vi "Transform Points using Homography Matrix.vi"(10 "Homography Matrix":dbl[][](array[numeric]), 11 "Points":cluster{"X":dbl, "Y":dbl}[](array[cluster])) -> (3 "Transformed Points":cluster{"X":dbl, "Y":dbl}[](array[cluster]))   [LabVIEW 2016]
doc: "The VI transforms the given array of points using the homography matrix.\n[x'] = [H] * [x]"
uses:
  <vilib>/Analysis/baseanly.llb/A x Vector.vi
  <vilib>/Analysis/NI_AALBase.lvlib
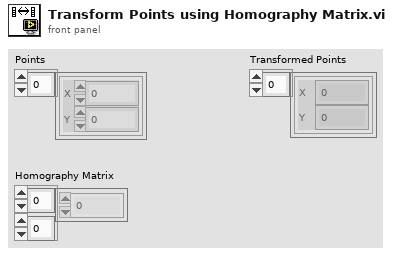
[diagram p1: front panel]
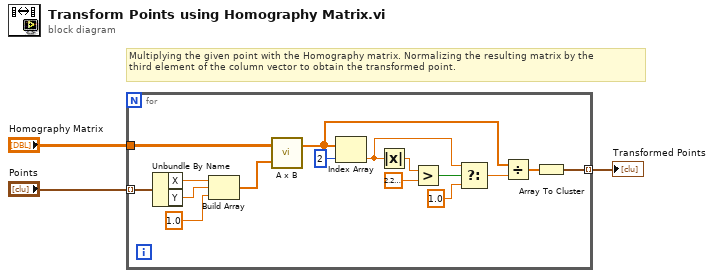
[diagram p0: block diagram]
diagram:
  # "Multiplying the given point with the Homography matrix. Normalizing the resulting matrix by the \nthird element of the column vector to obtain the transformed point."
  n1 = for {
    tunnel: "Homography Matrix" -> [w19]
    tunnel: "Points" -> [w12] mode=indexing
    tunnel: [w4] -> w2 mode=indexing
    n2 = Unbundle By Name(w12) -> ("X"=w11:dbl, "Y"=w10:dbl)
    n3 = Build Array(w11, w10, 1.0) -> (w13:dbl[])
    n4 = call-poly <vilib>:"A x B.vi"("Vector"=w13, "A"=w19) -> ("A x Vector"=w16:dbl[])  [unwired: 1 out]
    n5 = Index Array(array=w16, index=2) -> (element=w8:dbl)
    n6 = Absolute Value(x=w8) -> (abs(x)=w17:dbl)
    n7 = Greater?(x=w17, y=2.220446049250313e-16) -> (0:w9:bool)
    n8 = Select(t=w8, s=w9, f=1.0) -> (s? t:f=w6:dbl)
    n9 = Divide(x=w16, y=w6) -> (x/y=w5:dbl[])
    n10 = Array To Cluster(array=w5) -> (cluster=w4:cluster{"[0]":dbl, "[1]":dbl})
  }
  "Transformed Points" <- w2
